vi "coutoutALL.vi"(6 "value":dbl, 8 "error in (no error)":errorcluster caption="错误输入（无错误）", 9 "value 2":dbl, 10 "Value":bool[](array[boolean]), 11 "MulticolumnListbox输入":refnum<vi>) -> (0 "error out":errorcluster caption="错误输出", 1 "NG输出":dbl, 2 "OK输出":dbl, 3 "总数输出":dbl, 4 "良率":dbl)   [LabVIEW 2018]
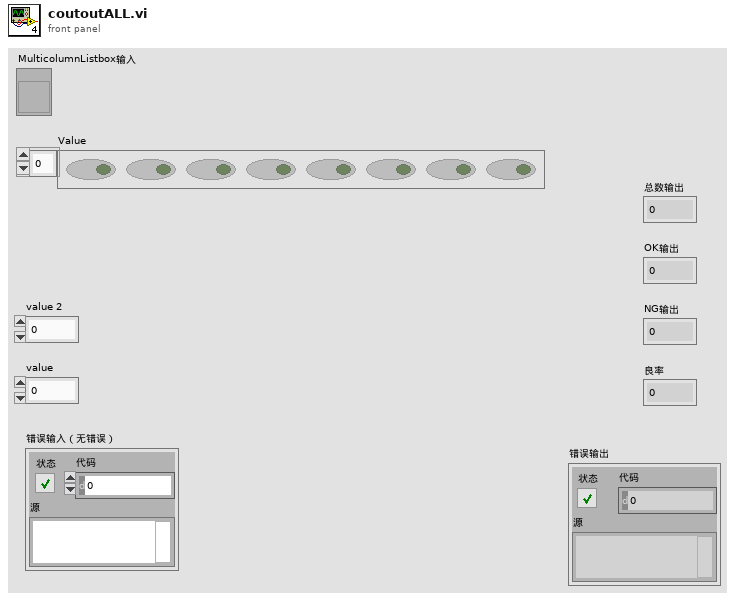
[diagram p1: front panel]
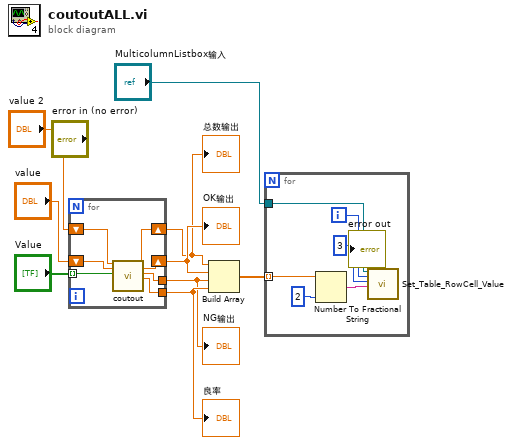
[diagram p0: block diagram]
diagram:
  n1 = for {
    tunnel: "Value" -> [w16] mode=indexing
    tunnel: [w13] -> w6
    tunnel: [w12] -> w7
    shift-right: [w15] -> w4
    shift-left: "value 2" -> [w11]
    shift-right: [w14] -> w5
    shift-left: "value" -> [w10]
    n2 = call "coutout.vi"("总数输入"=w11, "OK输入"=w10, "OK"=w16) -> ("总数输出"=w15:dbl, "OK输出"=w14:dbl, "NG输出"=w13:dbl, "良率"=w12:dbl)  [unwired: 12 in, 1 out]
  }
  "良率" <- w7
  "NG输出" <- w6
  "OK输出" <- w5
  "总数输出" <- w4
  n3 = Build Array(w4, w5, w6, w7) -> (w8:dbl[])
  n4 = for {
    tunnel: w8 -> [w19] mode=indexing
    tunnel: "MulticolumnListbox输入" -> [w17]
    i -> [w21]
    n5 = Number To Fractional String(number=w19, precision (6)=i16 2 ("精度(6)")) -> (F-format string=w18:string)  [unwired: 2 in]
    n6 = call "Set_Table_RowCell_Value.vi"("测试信息 2"=w17, "索引 (行)"=w21, "禁用的索引 (列)"=3, "新元素/子数组"=w18) -> ()  [unwired: 14 in, 2 out]
  }
